vi "Toggle Latch.vi"(11 "Clamp Toggled?":bool=TRUE) -> (3 "Clamp Toggled":bool=TRUE)   [LabVIEW 2014]
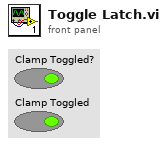
[diagram p1: front panel]
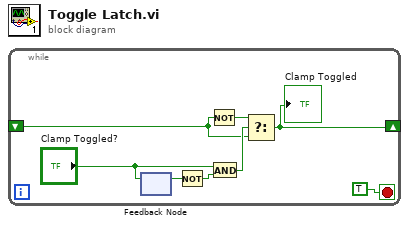
[diagram p0: block diagram]
diagram:
  n1 = while {
    shift-right: [w2] -> _
    shift-left: _ -> [w1]
    stop <- TRUE stop-if-true
    n2 = feedback-in #1("Clamp Toggled?") -> ()
    n3 = feedback #1() -> (w6:bool)  [unwired: 1 in]
    n4 = Not(x=w6) -> (.not. x?=w5:bool)
    n5 = Not(x=w1) -> (.not. x?=w3:bool)
    n6 = And(x="Clamp Toggled?", y=w5) -> (x .and. y?=w4:bool)
    n7 = Select(t=w3, s=w4, f=w1) -> (s? t:f=w2:bool)
    "Clamp Toggled" <- w2
  }
